vi "oa_Attach Elapsed Time Info.vi"(7 "reset? (F)":bool, 8 "error in (no error)":errorcluster, 9 "time/speed segment [s or rpm]":cluster{"start":dbl, "end":dbl, "step size":dbl} {"step size" format="%.2f"; "end" min=0.0 format="%.2f"; "start" min=0.0 format="%.2f"}, 10 "plot type":T1(ring), 11 "scaled signal [EU]":waveform(dbl)={"t0"=timestamp(0 s since 1904-01-01), "dt"=0.0, "Y"=[]}) -> (0 "error out":errorcluster, 3 "scaled signal [EU] out":waveform(dbl))   [LabVIEW 2017, in "SoundVib_Resampling.lvlib"]
uses:
  <vilib>/addons/Sound and Vibration/Order Analysis/Resample Order Tracking/SoundVib_Resampling.lvlib
  <vilib>/Waveform/WDTOps.llb/WDT Waveform Duration DBL.vi
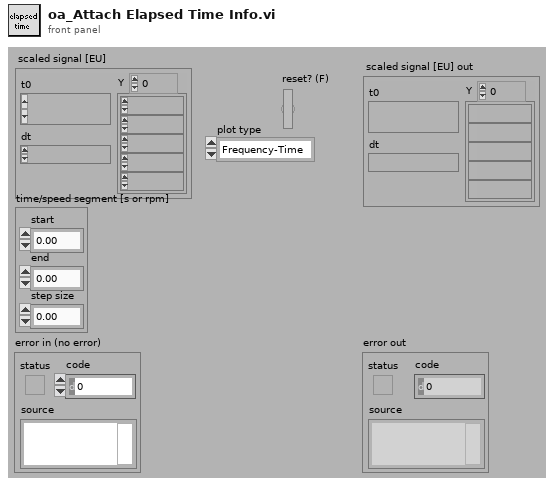
[diagram p1: front panel]
types:
  T1 = enum16{"Frequency-Time", "Time-Frequency", "Order-Time", "Time-Order", "Frequency-RPM", "RPM-Frequency", "Order-RPM", "RPM-Order"}
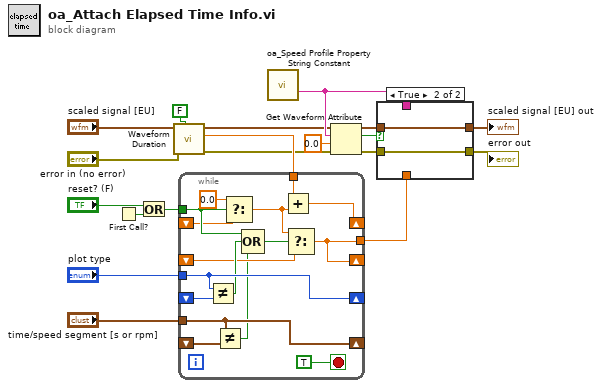
[diagram p0: block diagram]
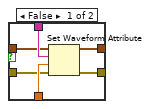
[diagram p2: hidden frame]
diagram:
  n1 = First Call?() -> (First Call?: T/F=w18:bool)
  n2 = Or(x="reset? (F)", y=w18) -> (x .or. y?=w17:bool)
  n3 = call-poly <vilib>:"Waveform Duration.vi"("open interval? (T)"=FALSE, "error in (no error)"="error in (no error)", "waveform in"="scaled signal [EU]") -> ("error out"=w7:errorcluster, "duration"=w10:dbl, "waveform out"=w6:waveform(dbl))  [unwired: 6 in]
  n4 = while {
    tunnel: w10 -> [w28]
    tunnel: w17 -> [w30]
    shift-right: [w33] -> _
    shift-left: _ -> [w26]
    tunnel: "plot type" -> [w32]
    shift-right: [w32] -> _
    shift-left: _ -> [w31]
    shift-right: [w24] -> _
    shift-left: _ -> [w25]
    tunnel: [w24] -> w9
    shift-right: [w21] -> _
    shift-left: _ -> [w22]
    tunnel: "time/speed segment [s or rpm]" -> [w21]
    stop <- TRUE stop-if-true
    n5 = Not Equal?(x=w32, y=w31) -> (x != y?=w29:bool)
    n6 = Not Equal?(x=w21, y=w22) -> (x != y?=w20:bool)
    n7 = Select(t=0.0, s=w30, f=w26) -> (s? t:f=w23:dbl)
    n8 = Compound Arithmetic op=OR(w30, w29, w20) -> (w27:bool)
    n9 = Add(x=w28, y=w23) -> (x+y=w33:dbl)
    n10 = Select(t=w23, s=w27, f=w25) -> (s? t:f=w24:dbl)
  }
  n11 = call <vilib>:"oa_Speed Profile Property String Constant.vi"() -> ("elapsed time"=w8:string)  [unwired: 12 in, 3 out]
  n12 = Get Waveform Attribute(4:w7, 5:0.0, 6:w8, 7:w6) -> (0:w2:errorcluster, 2:w3:bool, 3:w5:waveform(dbl))  [unwired: 1 out]
  n13 = case shown="True" w3 {
    tunnel: [w41 w42] -> w15
    tunnel: [w40 w43] -> w14
    tunnel: w9 -> [w39 _]
    tunnel: w8 -> [w38 _]
    tunnel: w5 -> [w37 w43]
    tunnel: w2 -> [w36 w42]
    frame False {
      n14 = Set Waveform Attribute(4:w36, 5:w39, 6:w38, 7:w37) -> (0:w41:errorcluster, 3:w40:waveform(dbl))  [unwired: 1 out]
    }
    frame True {
    }
  }
  "error out" <- w15
  "scaled signal [EU] out" <- w14
